vi "Add Value with TS.vi"(8 "Error In":errorcluster, 9 "Value":dbl, 10 "Time Stamp":timestamp format="%<%x %.3X>T", 11 "BNT_XtGraph in":refnum<class "BNT_XtGraph.lvclass">) -> (0 "Error Out":errorcluster, 3 "BNT_XtGraph out":refnum<class "BNT_XtGraph.lvclass">)   [LabVIEW 2019, in "BNT_XtGraph.lvlib" / "BNT_XtGraph.lvclass"]
doc: "Add actual value with timestamp to history."
uses:
  BNT_XtGraph.lvclass
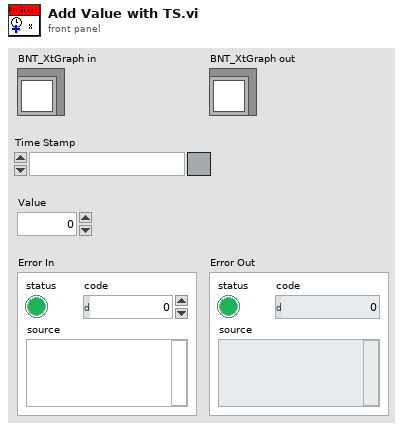
[diagram p1: front panel]
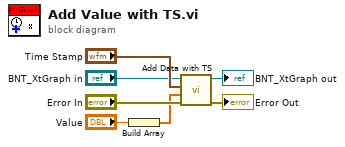
[diagram p0: block diagram]
diagram:
  n1 = Build Array("Value") -> (w1:dbl[])
  n2 = call "Add Data with TS.vi"("Error In"="Error In", "Values"=w1, "Time Stamp"="Time Stamp", "BNT_XtGraph in"="BNT_XtGraph in") -> ("Error Out"=→"Error Out":errorcluster, "BNT_XtGraph out"=→"BNT_XtGraph out":refnum<class "BNT_XtGraph.lvclass">)  [unwired: 6 in]
